vi "TcA03-006_ClassAttributesCanBeUnlockedWithoutBeingModified.vi"(1 "Input buffer":T3="1", 3 "Invocation info":T2, 5 "error in (no error)":errorcluster, 6 "Add log to result?":bool) -> (16 "Test Data":T1 {"Numeric Measurement" format="%.2f"}, 19 "error out":errorcluster)   [LabVIEW 2020]
doc: "Test case template."
uses:
  Shared/Support_InputBuffer.ctl
  Shared/Support_InvocationInfo.ctl
  Shared/Support_TestData.ctl
  TestClasses/G#BaseClass2_class/G#BaseClass2.lvclass
  TestClasses/G#SubClass2_class/G#SubClass2.lvclass
  <vilib>/addons/_AddQ/G#Object/G#Object.lvclass
panel:
  in  "Test name":string="TcA03-006 Class attributes can be unlocked without being modified"
  out "Test result":bool
  out "Result":string
  # "Verify that class attributes can be unlocked without being\nmodified if an error occurs while modifying or forced to be unlocked."
  # "Sub test case"
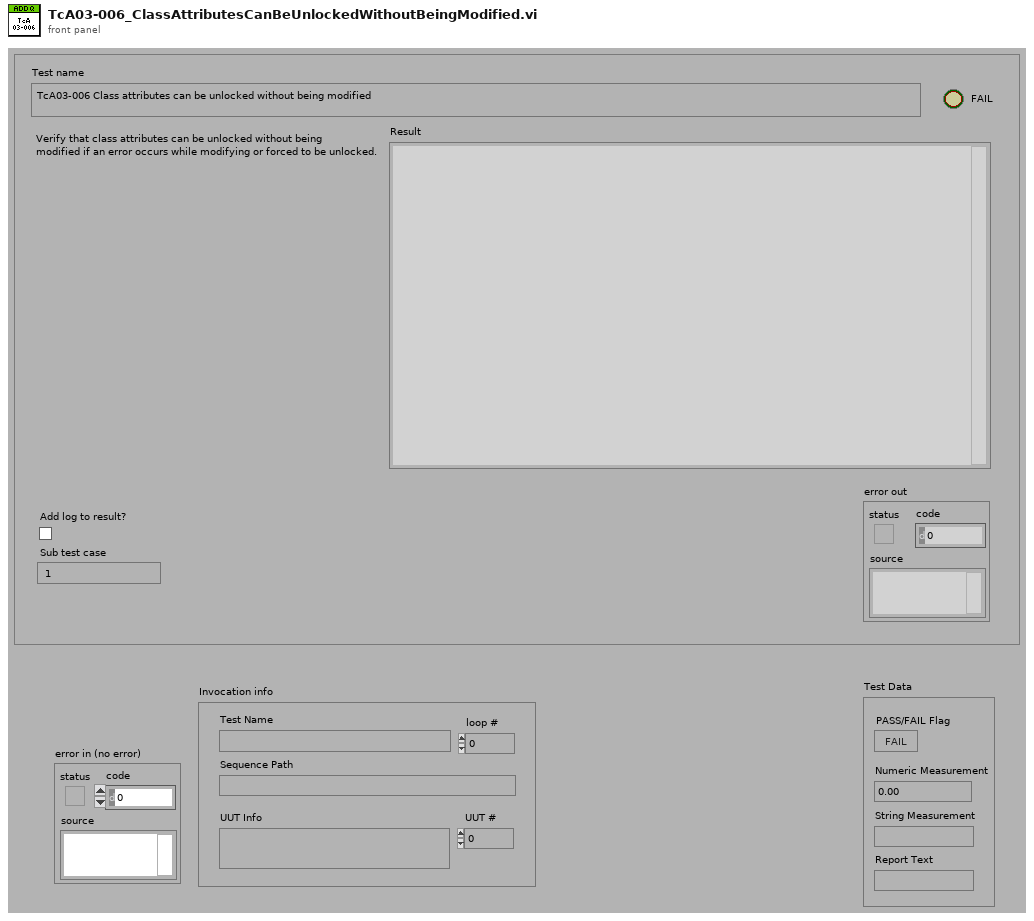
[diagram p1: front panel]
types:
  T1 = typedef "Support_TestData.ctl" = cluster{"PASS/FAIL Flag":bool, "Numeric Measurement":dbl, "String Measurement":string, "Report Text":string}
  T2 = typedef "Support_InvocationInfo.ctl" = cluster{"UUT #":i32, "loop #":i32, "UUT Info":string, "Test Name":string, "Sequence Path":path}
  T3 = typedef "Support_InputBuffer.ctl" = string
  T4 = typedef "Support_ResultType.ctl" = cluster{"Pass":bool, "Comment":string, "MeasurementValue":dbl}
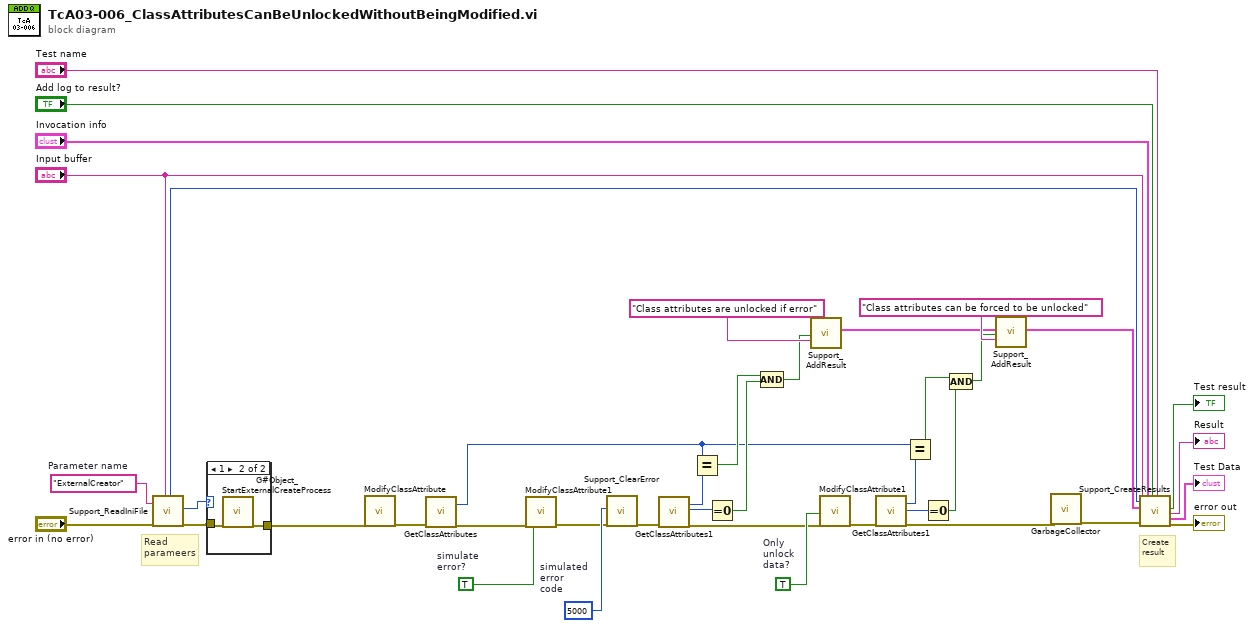
[diagram p0: block diagram]
diagram:
  w1 = "ExternalCreator"  # Parameter name
  w24 = TRUE  # Only unlock data?
  w26 = 5000  # simulated error code
  w12 = TRUE  # simulate error?
  # "Create\nresult"
  # "Read\nparameers"
  n1 = call "Support_ReadIniFile.vi"("Parameter name"=w1, "error in (no error)"="error in (no error)", "Sub test case"="Input buffer") -> ("Timer start"=w31:u32, "Parameter1 as I32"=w3:i32, "error out"=w4:errorcluster)  [unwired: 9 in, 5 out]
  n2 = case shown="1" w3 {
    tunnel: w4 -> [w41 w43]
    tunnel: [w41 w42] -> w2
    frame 0, Default {
    }
    frame 1 {
      n3 = call <vilib>:"G#Object_StartExternalCreateProcess.vi"("error in (no error)"=w43) -> ("error out"=w42:errorcluster)  [unwired: 18 in]
    }
  }
  n4 = call "ModifyClassAttribute.vi"("error in (no error)"=w2) -> ("error out"=w28:errorcluster)  [unwired: 16 in, 2 out]
  n5 = call "GetClassAttributes.vi"("error in (no error)"=w28) -> ("ClassAttr"=w5:i32, "error out"=w27:errorcluster)  [unwired: 16 in, 1 out]
  n6 = call "ModifyClassAttribute1.vi"("error in (no error)"=w27, "status"=w12) -> ("error out"=w20:errorcluster)  [unwired: 15 in, 2 out]
  n7 = call "Support_ClearError.vi"("code"=w26, "error in (no error)"=w20) -> ("error out"=w19:errorcluster)  [unwired: 16 in, 1 out]
  n8 = call "GetClassAttributes1.vi"("error in (no error)"=w19) -> ("Base class.ClassAttr"=w11:i32, "SubClassAttr"=w10:i32, "error out"=w18:errorcluster)  [unwired: 15 in, 1 out]
  n9 = Equal?(x=w5, y=w11) -> (x = y?=w17:bool)
  n10 = Equal To 0?(x=w10) -> (x = 0?=w9:bool)
  n11 = Compound Arithmetic op=AND(w17, w9) -> (w16:bool)
  n12 = call "Support_AddResult.vi"("Pass"=w16, "Comment"="Class attributes are unlocked if error") -> ("Results out"=w22:T4[])  [unwired: 17 in]
  n13 = call "ModifyClassAttribute1.vi"("Only unlock data? (F)"=w24, "error in (no error)"=w18) -> ("error out"=w25:errorcluster)  [unwired: 15 in, 2 out]
  n14 = call "GetClassAttributes1.vi"("error in (no error)"=w25) -> ("Base class.ClassAttr"=w8:i32, "SubClassAttr"=w7:i32, "error out"=w13:errorcluster)  [unwired: 15 in, 1 out]
  n15 = Equal?(x=w5, y=w8) -> (x = y?=w15:bool)
  n16 = Equal To 0?(x=w7) -> (x = 0?=w6:bool)
  n17 = Compound Arithmetic op=AND(w15, w6) -> (w14:bool)
  n18 = call "Support_AddResult.vi"("Results in"=w22, "Pass"=w14, "Comment"="Class attributes can be forced to be unlocked") -> ("Results out"=w21:T4[])  [unwired: 16 in]
  n19 = call <vilib>:"GarbageCollector.vi"("error in (no error)"=w13) -> ("error out"=w30:errorcluster)  [unwired: 16 in, 2 out]
  n20 = call "Support_CreateResults.vi"("Sub test case"="Input buffer", "Timer start"=w31, "Results"=w21, "error in (no error)"=w30, "Invocation info"="Invocation info", "Add log to result?"="Add log to result?", "Test name"="Test name") -> ("Pass/fail flag"=→"Test result":bool, "Result"=→"Result":string, "Test Data"=→"Test Data":T1, "error out"=→"error out":errorcluster)  [unwired: 9 in]
